vi "(Depricated) Sample In.vi"(8 "error in (no error)":errorcluster, 10 "Sample":refnum<class "Sample.lvclass">, 11 "Transfer Line in":refnum<class "Transfer Line.lvclass">) -> (0 "error out":errorcluster, 3 "Transfer Line out":refnum<class "Transfer Line.lvclass">)   [LabVIEW 2014]
uses:
  Transfer Line.lvclass
  subs/Sample/Sample.lvclass
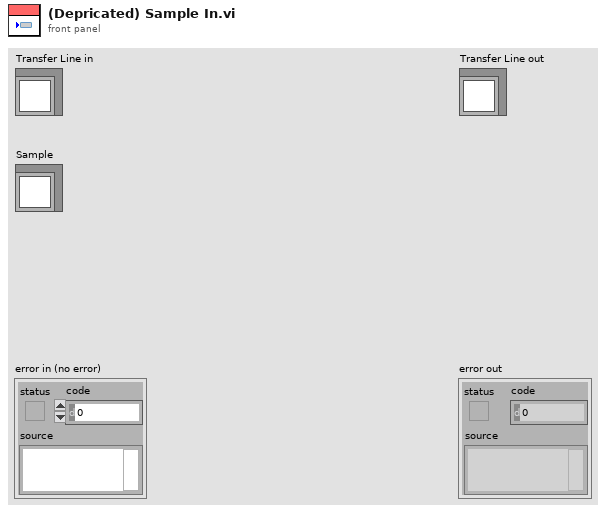
[diagram p1: front panel]
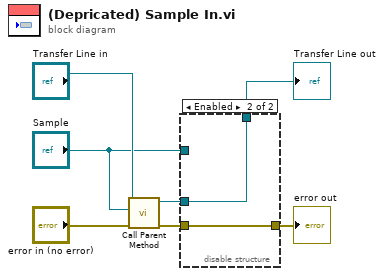
[diagram p0: block diagram]
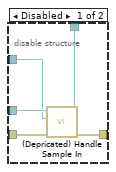
[diagram p2: hidden frame]
diagram:
  n1 = call-parent "Call Parent Method"("error in (no error)"="error in (no error)", "Sample"="Sample", "CO2 Actor in"="Transfer Line in") -> ("error out"=w5:errorcluster, "CO2 Actor out"=w4:refnum<class "Transfer Line.lvclass">)  [unwired: 7 in]
  n2 = disable-structure shown="Enabled" {
    disable-tunnel: w5 -> [w12 w13]
    disable-tunnel: w4 -> [w11 w14]
    disable-tunnel: [w10 w13] -> w3
    disable-tunnel: [w9 w14] -> w2
    disable-tunnel: "Sample" -> [w8 _]
    frame Disabled {
      n3 = call "(Depricated) Handle Sample In.vi"("error in (no error)"=w12, "Sample"=w8, "Transfer Line in"=w11) -> ("error out"=w10:errorcluster, "Transfer Line out"=w9:refnum<class "Transfer Line.lvclass">)  [unwired: 7 in]
    }
    frame Enabled {
    }
  }
  "error out" <- w3
  "Transfer Line out" <- w2
